vi "Process.vi"(8 "error in":errorcluster, 11 "Generator":refnum<class "Generator.lvclass">) -> (0 "error out":errorcluster, 3 "Generator out":refnum<class "Generator.lvclass">)   [LabVIEW 2019, in "Generator.lvclass"]
uses:
  Generator.lvclass
  C:/Program Files/National Instruments/LabVIEW 2019/vi.lib/JKI/JKI SMO/SMO/SMO.lvclass
  Generator.lvclass/Generator.ctl
  typedefs/Generator.State--enum.ctl
  <vilib>/JKI/JKI SMO/SMO/SMO.lvclass/SMO.ctl
  929f499e-e52d-49ce-8fd4-6eb7de19c2ac.vi
  9c9ff3dc-a17c-4e79-91bb-522cf085dd97.vi
  7f9fb2fb-b452-4165-b08b-fdce49342378.vi
  <vilib>/JKI/JKI SMO/SMO/Private/ReftoDVR--SMO.vi
  <vilib>/dlg_ctls.llb/Space Constant.vi
  <vilib>/AdvancedString/1D String Array to Delimited String.vi
  <vilib>/JDP Science/JSONtext/Variant to JSON Text.vi
  <vilib>/JDP Science/JSONtext/LVClass Serializer/JSONtext LVClass Serializer.lvclass
  <vilib>/JKI/JKI SMO/SMO/SMO.lvclass
  <userlib>/LevyLab/Debug/Debug.lvlib
panel:
  out "time (ms)":dbl=1.0 min=1.0 format="%#_6p"
  out "String 3":string
  in  "timeout (ms)":i32=10 min=1
  out "String 2":string
  out "String":string
  # "Generator"
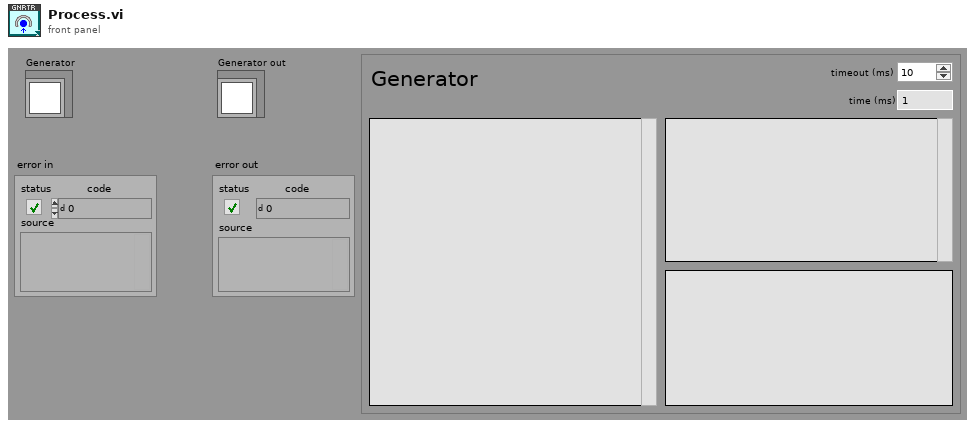
[diagram p1: front panel]
types:
  T1 = typedef "Generator.lvclass/Generator.State--enum.ctl" = enum16{"idle", "started"}
  T2 = enum32{"invalid app kind", "Development System", "Run Time System", "Student Edition", "Embedded LabVIEW", "Evaluation", "Custom"}
  T3 = enum32{"Invalid", "Standard", "Closed", "Hidden", "Minimized", "Maximized"}
  T4 = cluster{"Core":cluster{"Current VI Reference":refnum<vi>, "Close Panel on Exit?":bool, "Last Error":cluster{"error":errorcluster, "previous state":string, "remaining states":string}, "Shutdown?":bool}, "SMO":refnum<class "Generator.lvclass">, "state":T1}
  T5 = typedef "Generator.lvclass/AO.Channel--Cluster--Array.ctl" = T6[]
  T6 = typedef "Generator.lvclass/AO.Channel--Cluster.ctl" = cluster{"Enable?":bool, "Channel":i32, "Amplitude":dbl, "Offset":dbl, "Frequency":dbl, "Phase":dbl, "Function":T7, "Sweeping?":bool, "Limit AC?":bool, "Limit DC?":bool, "Duty Cycle?":bool, "Duty Cycle":dbl}
  T7 = typedef "Generator.lvclass/AO.Channel.Function--Enum.ctl" = enum16{"sine", "square", "triangle", "saw"}
  T8 = typedef "Generator.lvclass/REF.Channel--Cluster--Array.ctl" = T9[]
  T9 = typedef "Generator.lvclass/REF.Channel--Cluster.ctl" = cluster{"Enable?":bool, "Channel":i32, "Frequency":dbl, "Phase":dbl, "TC":dbl, "Roll-Off":i32}
  T10 = typedef "Generator.lvclass/Sweep.Channel--Cluster--Array.ctl" = T11[]
  T11 = typedef "Generator.lvclass/Sweep.Channel--Cluster.ctl" = cluster{"Enable?":bool, "Channel":u16, "Start":dbl, "End":dbl, "Pattern":T12, "Table":dbl[]}
  T12 = typedef "Generator.lvclass/Sweep.Pattern--Enum.ctl" = enum16{"Ramp /", "Ramp /\\", "Smooth Ramp _/", "Smooth Ramp _/\\_", "Table"}
  T13 = typedef "Generator.lvclass/Generator.Command--enum.ctl" = enum16{"start", "stop", "start sweep", "stop sweep"}
  T14 = cluster{"Current VI Reference":refnum<vi>, "Close Panel on Exit?":bool, "Last Error":cluster{"error":errorcluster, "previous state":string, "remaining states":string}, "Shutdown?":bool}
  T15 = typedef "Debug.lvlib/Attribute.Debug.lvclass/DebugBehavior.ctl" = enum16{"Normal", "Debug"}
  T16 = typedef "SMO.lvclass/Protected Events.ctl" = cluster{"StopProcesses":refnum<user-event>, "AbortProcesses":refnum<user-event>, "Config Changed":refnum<user-event>, "Dependency":refnum<user-event>}
  T17 = typedef "Generator.lvclass/PrivateEvents--Cluster.ctl" = cluster{"Message":refnum<user-event>, "Sampling":refnum<user-event>, "AOchannel":refnum<user-event>, "REFchannel":refnum<user-event>, "Sweep":refnum<user-event>, "Command":refnum<user-event>, "WaveformQueues":refnum<user-event>}
  T18 = typedef "Generator.lvclass/Waveforms--Cluster.ctl" = cluster{"AO":waveform(dbl)[], "REF_X":waveform(dbl)[], "REF_Y":waveform(dbl)[]}
  T19 = typedef "Generator.lvclass/Generator.Sweep Status--enum.ctl" = enum16{"idle", "initializing", "waiting", "sweeping", "stopping"}
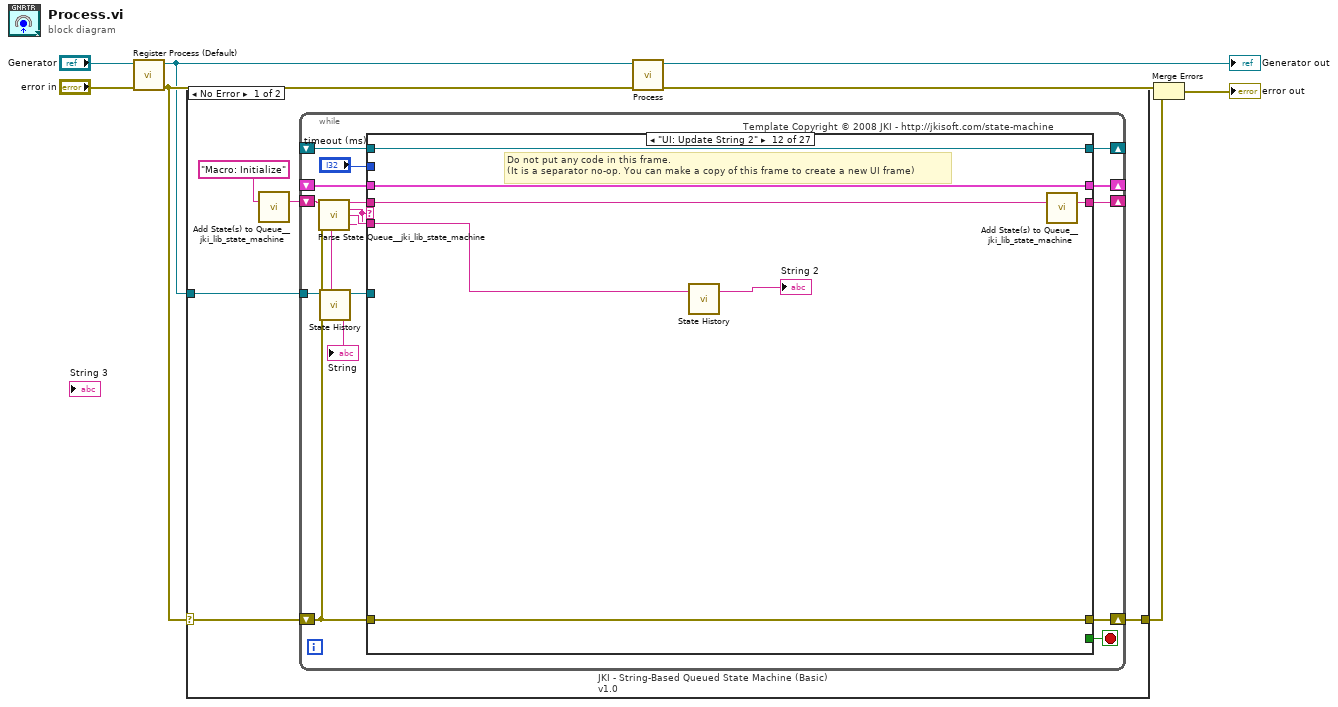
[diagram p0: block diagram]
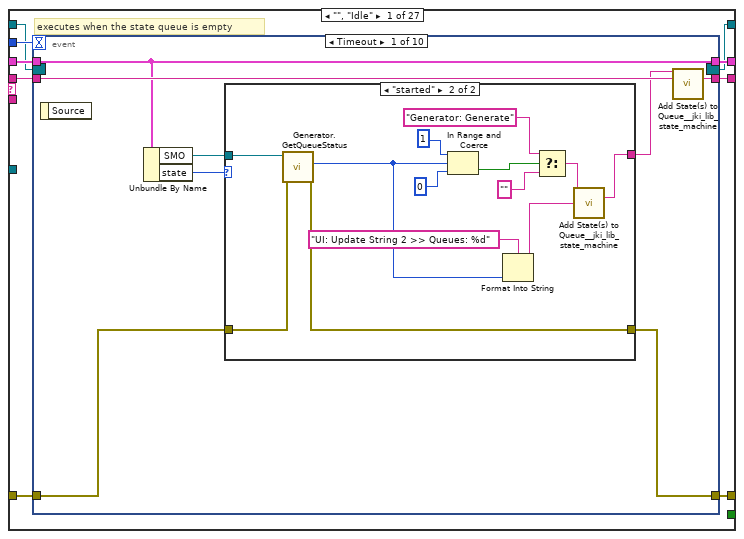
[diagram p2: hidden frame]
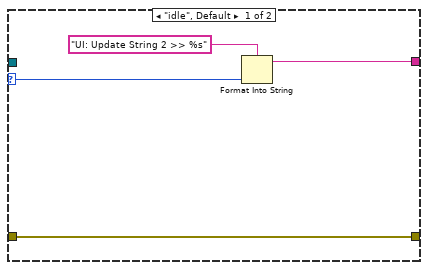
[diagram p3: hidden frame]
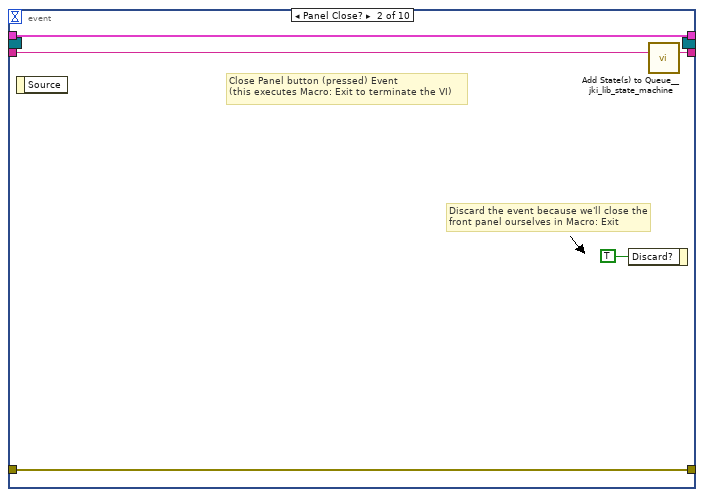
[diagram p4: hidden frame]
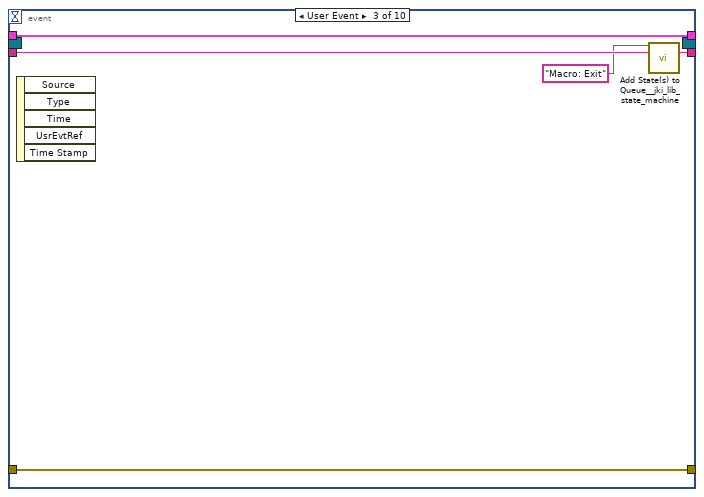
[diagram p5: hidden frame]
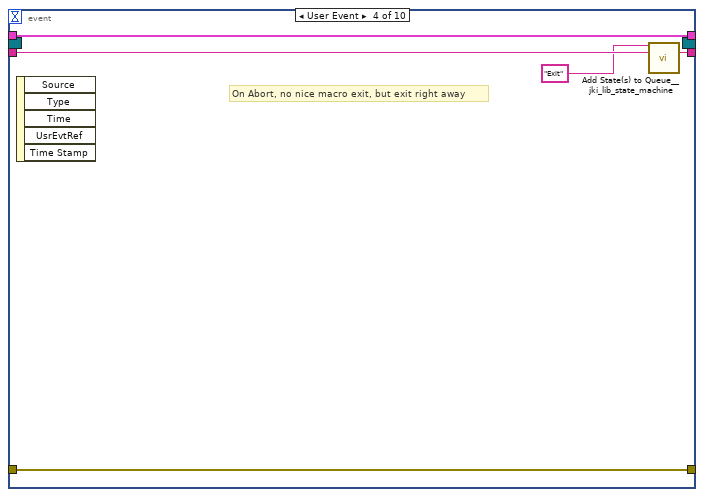
[diagram p6: hidden frame]
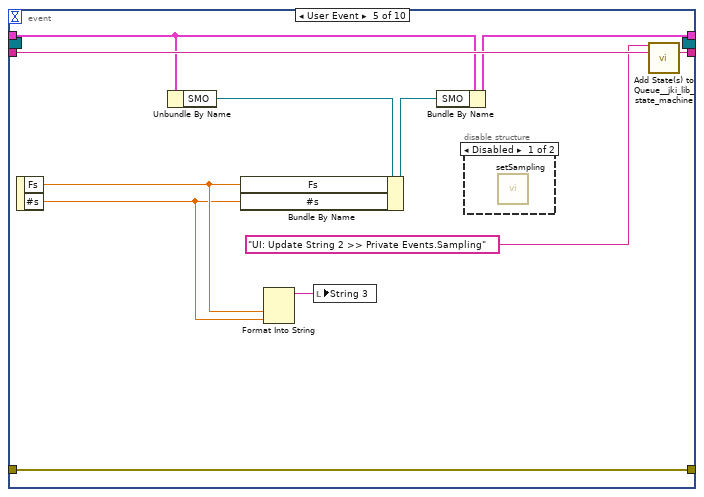
[diagram p7: hidden frame]
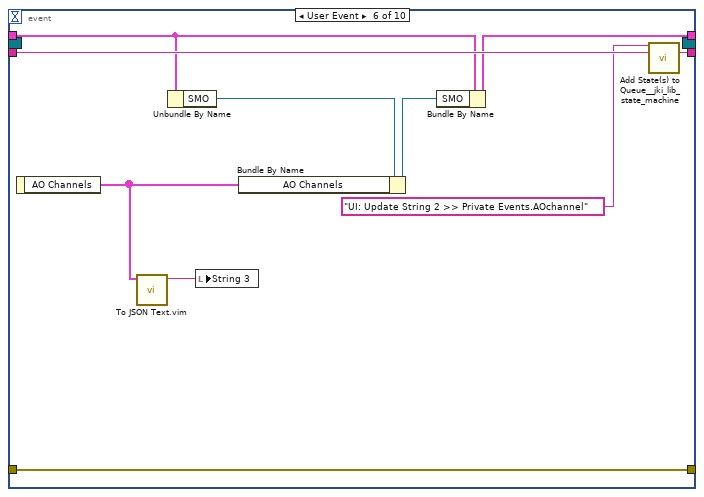
[diagram p9: hidden frame]
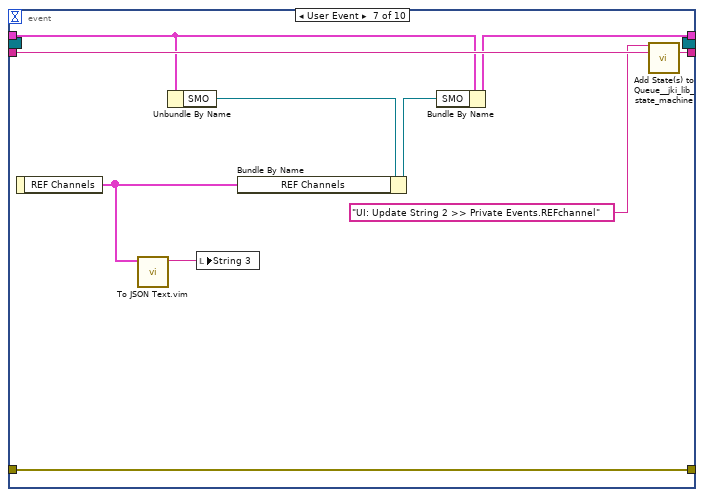
[diagram p10: hidden frame]
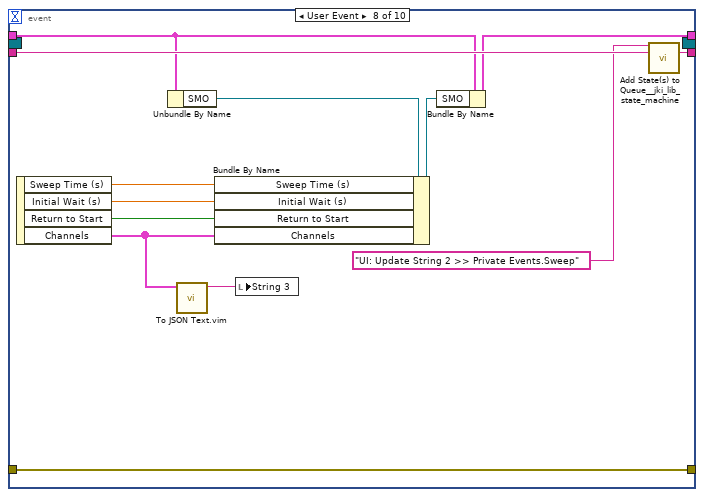
[diagram p11: hidden frame]
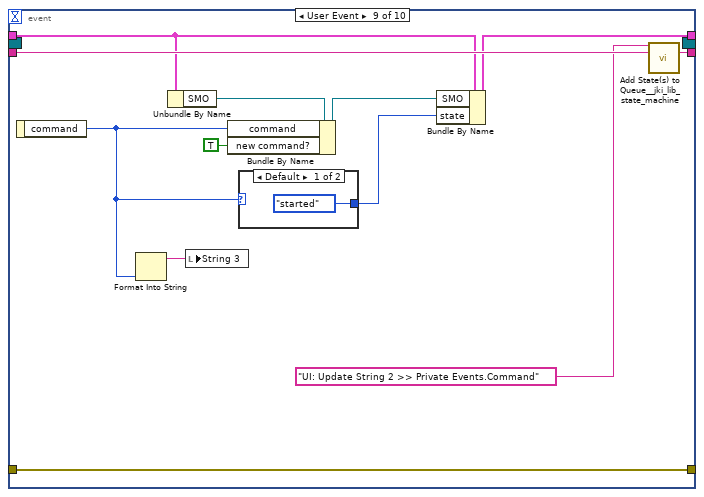
[diagram p12: hidden frame]
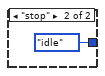
[diagram p13: hidden frame]
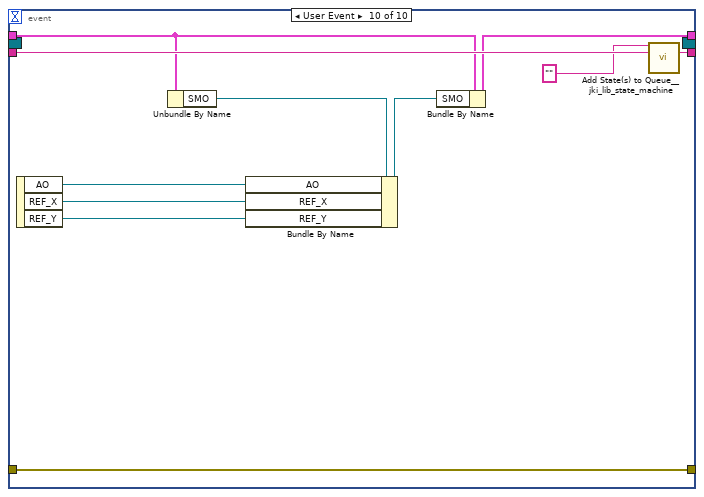
[diagram p14: hidden frame]
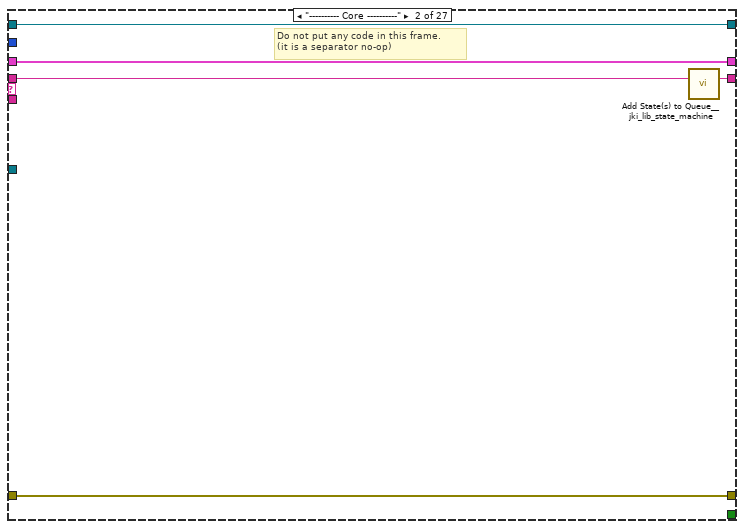
[diagram p15: hidden frame]
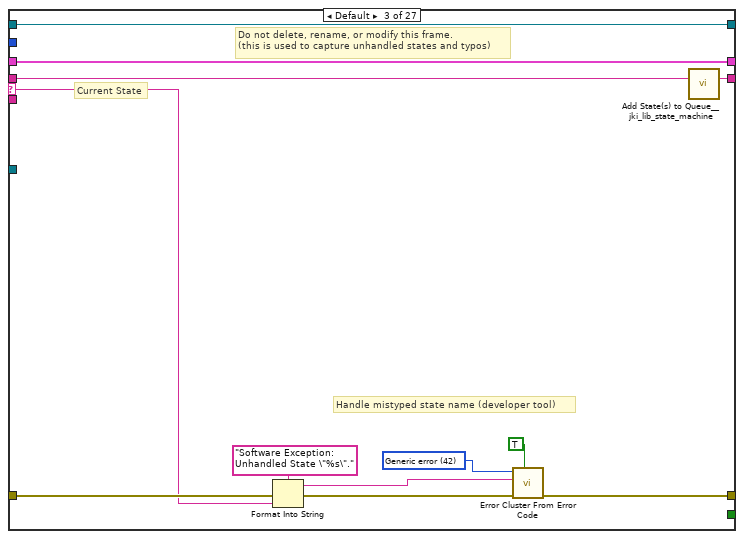
[diagram p16: hidden frame]
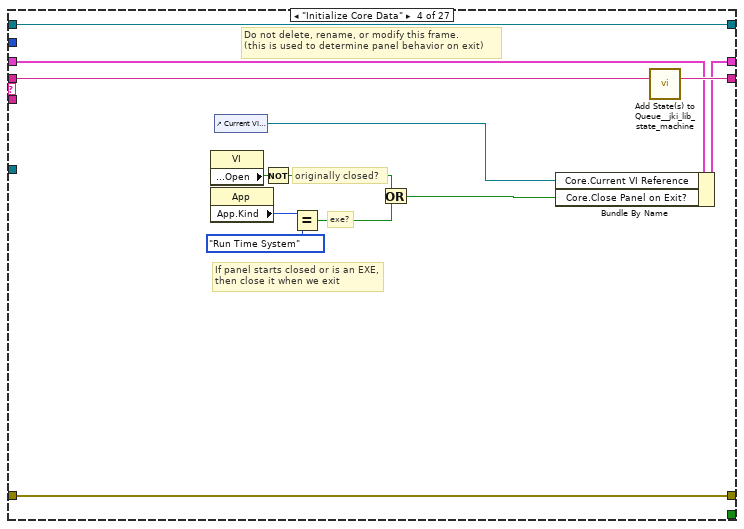
[diagram p17: hidden frame]
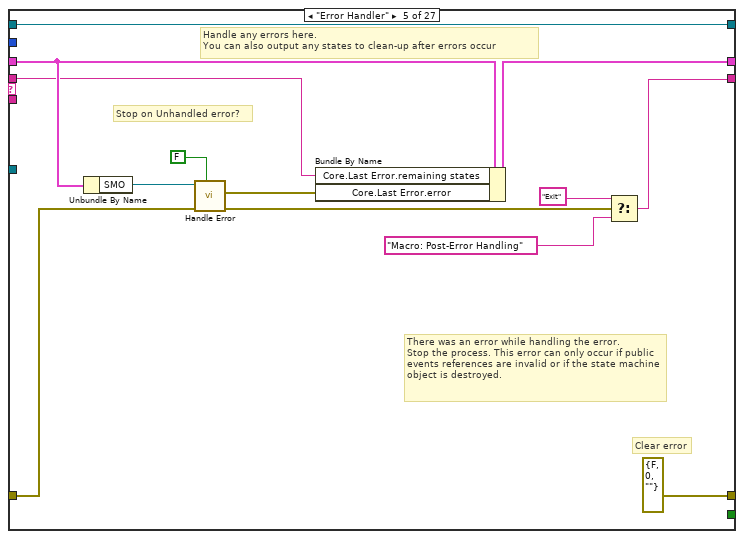
[diagram p18: hidden frame]
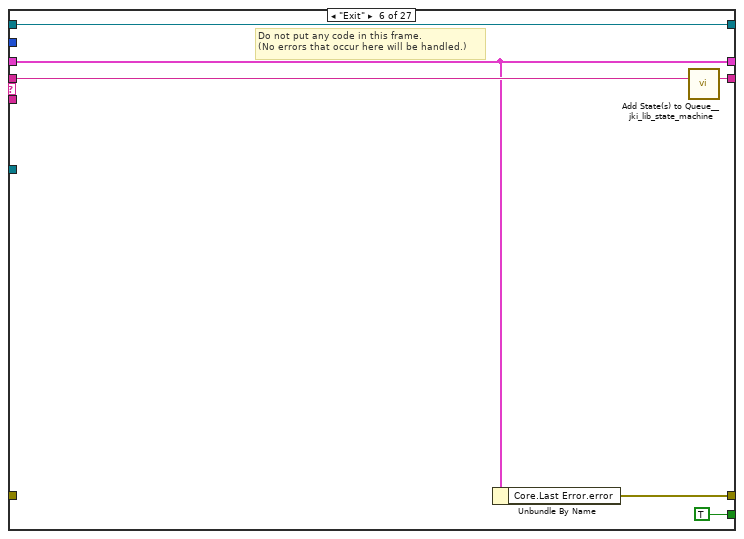
[diagram p19: hidden frame]
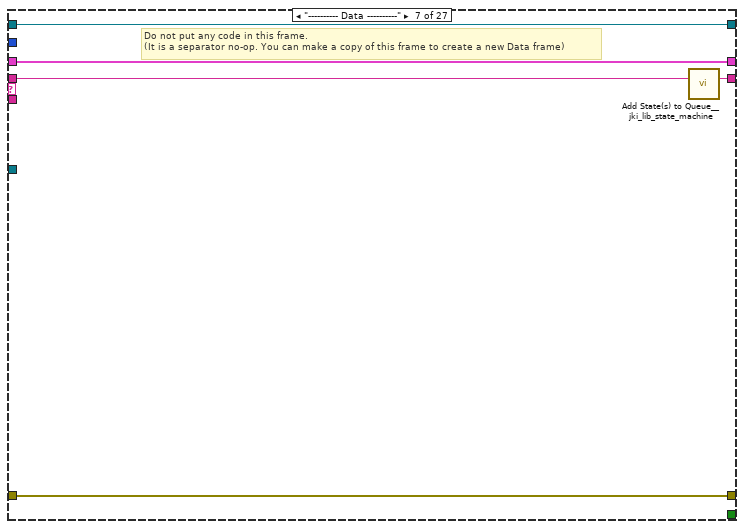
[diagram p20: hidden frame]
diagram:
  n1 = call <vilib>:"Register Process (Default).vi"("error in (no error)"="error in", "SMO"="Generator") -> ("error out"=w4:errorcluster, "SelfRef"=w3:refnum<class "Generator.lvclass">)  [unwired: 8 in]
  n2 = case shown="No Error" w4 {
    selector: w4 -> [w12 w441]
    tunnel: w3 -> [w13 _]
    tunnel: [w11 w441] -> w2
    frame No Error {
      n3 = call <vilib>:"Add State(s) to Queue__jki_lib_state_machine.vi"("State(s) in (\"\")"="Macro: Initialize") -> ("States Out"=w9:string)  [unwired: 14 in]
      n4 = while "JKI - String-Based Queued State Machine (Basic) v1.0" {
        shift-right: [w23] -> _
        shift-left: _ -> [w22]
        shift-right: [w26] -> w11
        shift-left: w12 -> [w21]
        shift-right: [w25] -> _
        shift-left: w9 -> [w27]
        tunnel: w13 -> [w16]
        shift-right: [w20] -> _
        shift-left: _ -> [w19]
        stop <- w24 stop-if-true
        # "Template Copyright © 2008 JKI - http://jkisoft.com/state-machine"
        n5 = call <vilib>:"Parse State Queue__jki_lib_state_machine.vi"("State Queue"=w27, "Error In (no error)"=w21) -> ("Remaining States"=w29:string, "Current State"=w15:string, "Arguments"=w28:string)  [unwired: 11 in]
        n6 = call <userlib>:"State History.vi"("Current State"=w15, "SMO"=w16) -> ("SMO"=w17:refnum<class "Generator.lvclass">, "History"=→"String":string)  [unwired: 8 in]
        n7 = case shown="\"UI: Update String 2\"" w15 {
          selector: w15 -> [_ _ w154 _ _ _ _ _ _ _ _ _ w238 _ _ _ _ _ _ _ _ _ _ _ _ _ _]
          tunnel: w29 -> [w38 w152 w158 w177 w179 w196 w201 w209 w216 w221 w227 w234 w237 w257 w273 w305 w314 w320 w346 w363 w368 w379 w384 w397 w403 w410 w430]
          tunnel: w28 -> [_ _ _ _ _ _ _ _ _ _ _ w228 w235 w251 w269 _ _ _ _ _ _ _ _ _ _ _ _]
          tunnel: w22 -> [w36 w149 w156 w168 w188 w192 w198 _ w211 w218 w225 w231 w248 w255 w271 w302 w310 w317 w338 w353 w365 w376 w381 w395 w401 w406 w423]
          tunnel: [w35 w150 w160 w174 errorcluster {"status"=FALSE, "code"=0, "source"=""} ("error out") w191 w199 w204 w212 w219 w223 w232 w249 w252 w266 w303 w312 w316 w344 w361 w366 w370 w382 w388 w399 w404 w424] -> w26
          tunnel: w21 -> [w34 w150 w159 w174 w185 _ w199 w204 w213 w219 w222 w232 w249 w253 w267 w303 w312 w315 w344 w361 w366 w371 w382 w391 w399 w404 w426]
          tunnel: [w37 w151 w157 w176 w178 w195 w200 w208 w215 w220 w226 w233 w250 w256 w272 w304 w313 w329 w345 w362 w367 w378 w383 w396 w402 w409 w429] -> w25
          tunnel: [_ _ _ _ _ TRUE _ _ _ _ _ _ _ _ _ _ _ _ _ _ _ _ _ _ _ _ _] -> w24
          tunnel: [w33 w149 w156 w175 w187 w192 w198 w207 w211 w218 w225 w231 w248 w255 w271 w302 w310 w318 w342 w352 w365 w376 w381 w395 w401 w407 w427] -> w23
          tunnel: "timeout (ms)" -> [w32 _ _ _ _ _ _ _ _ _ _ _ _ _ _ _ _ _ _ _ _ _ _ _ _ _ _]
          tunnel: w17 -> [_ _ _ _ _ _ _ w203 _ _ _ _ _ _ _ _ _ _ _ _ _ _ _ _ _ _ _]
          tunnel: [w30 w148 w153 w165 w190 w193 w197 w206 w210 w217 w224 w230 w247 w254 w270 w301 w311 w328 w343 w355 w364 w377 w380 w393 w400 w408 w428] -> w20
          tunnel: w19 -> [w31 w148 w153 w165 w190 w193 w197 w206 w210 w217 w224 w230 w247 w254 w270 w301 w311 w328 w343 w355 w364 w377 w380 _ w400 w408 w428]
          frame "", "Idle" {
            # "executes when the state queue is empty"
            n8 = event shown="[0] Timeout" {
              selector: w31 -> [_ _ _ _ _ _ _ _ _ _]
              dyn-events: [_ _ _ _ _ _ _ _ _ _] -> w30
              timeout: w32 -> [_ _ _ _ _ _ _ _ _ _]
              tunnel: w38 -> [w46 w68 w73 w78 w89 w99 w109 w122 w134 w147]
              tunnel: [w45 w67 w72 w77 w88 w98 w108 w121 w133 w146] -> w37
              tunnel: w36 -> [w44 w64 w70 w75 w83 w92 w103 w114 w127 w139]
              tunnel: [w40 w66 w71 w76 w87 w97 w107 w120 w132 w145] -> w35
              tunnel: w34 -> [w41 w66 w71 w76 w87 w97 w107 w120 w132 w145]
              tunnel: [w44 w64 w70 w75 w84 w93 w104 w115 w128 w140] -> w33
              event Timeout {
                n9 = event-data() -> ()  [unwired: 1 in, 1 out]
                n10 = Unbundle By Name(w44) -> ("SMO"=w43:refnum<class "Generator.lvclass">, "state"=w39:T1)
                n11 = case shown="\"started\"" w39 {
                  selector: w39 -> [w49 _]
                  tunnel: w43 -> [_ w63]
                  tunnel: [w47 w52] -> w42
                  tunnel: w41 -> [w50 w56]
                  tunnel: [w50 w55] -> w40
                  frame "idle", Default {
                    n12 = Format Into String(format string="UI: Update String 2 >> %s" ("f"), w49) -> (resulting string=w47:string)  [unwired: 2 in, 1 out]
                  }
                  frame "started" {
                    n13 = call "Generator.GetQueueStatus.vi"("error in (no error)"=w56, "Generator in"=w63) -> ("error out"=w55:errorcluster, "# elements"=w60:i32)  [unwired: 7 in, 1 out]
                    n14 = In Range and Coerce(upper limit=1 ("x"), x=w60, lower limit=0 ("x")) -> (In Range?=w59:bool)  [unwired: 1 out]
                    n15 = Format Into String(format string="UI: Update String 2 >> Queues: %d" ("f"), w60) -> (resulting string=w54:string)  [unwired: 2 in, 1 out]
                    n16 = Select(t="Generator: Generate", s=w59, f="") -> (s? t:f=w53:string)
                    n17 = call <vilib>:"Add State(s) to Queue__jki_lib_state_machine.vi"("State(s) in Front (\"\")"=w53, "State(s) at Back (\"\")"=w54) -> ("States Out"=w52:string)  [unwired: 13 in]
                  }
                }
                n18 = call <vilib>:"Add State(s) to Queue__jki_lib_state_machine.vi"("State(s) in Front (\"\")"=w42, "State(s) in (\"\")"=w46) -> ("States Out"=w45:string)  [unwired: 13 in]
              }
              event Panel Close? {
                # "Discard the event because we'll close the front panel ourselves in Macro: Exit"
                # "Close Panel button (pressed) Event\n(this executes Macro: Exit to terminate the VI)"
                n19 = event-data() -> ()  [unwired: 1 in, 1 out]
                n20 = event-data("Discard?"=TRUE) -> ()  [unwired: 1 in, 1 out]
                n21 = call <vilib>:"Add State(s) to Queue__jki_lib_state_machine.vi"("State(s) in (\"\")"=w68) -> ("States Out"=w67:string)  [unwired: 14 in]
              }
              event User Event {
                n22 = event-data() -> ()  [unwired: 1 in, 5 out]
                n23 = call <vilib>:"Add State(s) to Queue__jki_lib_state_machine.vi"("State(s) in Front (\"\")"="Macro: Exit", "State(s) in (\"\")"=w73) -> ("States Out"=w72:string)  [unwired: 13 in]
              }
              event User Event {
                # "On Abort, no nice macro exit, but exit right away"
                n24 = event-data() -> ()  [unwired: 1 in, 5 out]
                n25 = call <vilib>:"Add State(s) to Queue__jki_lib_state_machine.vi"("State(s) in Front (\"\")"="Exit", "State(s) in (\"\")"=w78) -> ("States Out"=w77:string)  [unwired: 13 in]
              }
              event User Event {
                n26 = event-data() -> ("Fs"=w80:dbl, "#s"=w79:dbl)  [unwired: 1 in]
                n27 = Unbundle By Name(w83) -> ("SMO"=w86:refnum<class "Generator.lvclass">)
                n28 = Bundle By Name(cluster=w86, "Fs"=w80, "#s"=w79) -> (w85:refnum<class "Generator.lvclass">)
                n29 = Format Into String(w80, w79) -> (resulting string=w81:string)  [unwired: 3 in, 1 out]
                n30 = local write "String 3"(w81) -> ()
                n31 = Bundle By Name(cluster=w83, "SMO"=w85) -> (w84:T4)
                n32 = disable-structure shown="Disabled" {
                  frame Disabled {
                    n33 = call "setSampling.vi"() -> ()  [unwired: 10 in, 2 out]
                  }
                  frame Enabled {
                  }
                }
                n34 = call <vilib>:"Add State(s) to Queue__jki_lib_state_machine.vi"("State(s) in Front (\"\")"="UI: Update String 2 >> Private Events.Sampling", "State(s) in (\"\")"=w89) -> ("States Out"=w88:string)  [unwired: 13 in]
              }
              event User Event {
                n35 = event-data() -> ("AO Channels"=w91:T5)  [unwired: 1 in]
                n36 = call "To JSON Text.vim"("Anything"=w91) -> ("<JSON>"=w90:string)  [unwired: 9 in, 1 out]
                n37 = Unbundle By Name(w92) -> ("SMO"=w95:refnum<class "Generator.lvclass">)
                n38 = local write "String 3"(w90) -> ()
                n39 = Bundle By Name(cluster=w95, "AO Channels"=w91) -> (w94:refnum<class "Generator.lvclass">)
                n40 = Bundle By Name(cluster=w92, "SMO"=w94) -> (w93:T4)
                n41 = call <vilib>:"Add State(s) to Queue__jki_lib_state_machine.vi"("State(s) in Front (\"\")"="UI: Update String 2 >> Private Events.AOchannel", "State(s) in (\"\")"=w99) -> ("States Out"=w98:string)  [unwired: 13 in]
              }
              event User Event {
                n42 = event-data() -> ("REF Channels"=w100:T8)  [unwired: 1 in]
                n43 = call "To JSON Text.vim"("Anything"=w100) -> ("<JSON>"=w101:string)  [unwired: 9 in, 1 out]
                n44 = Unbundle By Name(w103) -> ("SMO"=w106:refnum<class "Generator.lvclass">)
                n45 = local write "String 3"(w101) -> ()
                n46 = Bundle By Name(cluster=w106, "REF Channels"=w100) -> (w105:refnum<class "Generator.lvclass">)
                n47 = Bundle By Name(cluster=w103, "SMO"=w105) -> (w104:T4)
                n48 = call <vilib>:"Add State(s) to Queue__jki_lib_state_machine.vi"("State(s) in Front (\"\")"="UI: Update String 2 >> Private Events.REFchannel", "State(s) in (\"\")"=w109) -> ("States Out"=w108:string)  [unwired: 13 in]
              }
              event User Event {
                n49 = event-data() -> ("Sweep Time (s)"=w118:dbl, "Initial Wait (s)"=w112:dbl, "Return to Start"=w113:bool, "Channels"=w110:T10)  [unwired: 1 in]
                n50 = Unbundle By Name(w114) -> ("SMO"=w117:refnum<class "Generator.lvclass">)
                n51 = call "To JSON Text.vim"("Anything"=w110) -> ("<JSON>"=w111:string)  [unwired: 9 in, 1 out]
                n52 = Bundle By Name(cluster=w117, "Sweep Time (s)"=w118, "Initial Wait (s)"=w112, "Return to Start"=w113, "Channels"=w110) -> (w116:refnum<class "Generator.lvclass">)
                n53 = local write "String 3"(w111) -> ()
                n54 = Bundle By Name(cluster=w114, "SMO"=w116) -> (w115:T4)
                n55 = call <vilib>:"Add State(s) to Queue__jki_lib_state_machine.vi"("State(s) in Front (\"\")"="UI: Update String 2 >> Private Events.Sweep", "State(s) in (\"\")"=w122) -> ("States Out"=w121:string)  [unwired: 13 in]
              }
              event User Event {
                n56 = event-data() -> ("command"=w124:T13)  [unwired: 1 in]
                n57 = Format Into String(w124) -> (resulting string=w125:string)  [unwired: 3 in, 1 out]
                n58 = Unbundle By Name(w127) -> ("SMO"=w130:refnum<class "Generator.lvclass">)
                n59 = local write "String 3"(w125) -> ()
                n60 = Bundle By Name(cluster=w130, "command"=w124, "new command?"=TRUE) -> (w129:refnum<class "Generator.lvclass">)
                n61 = case shown="Default" w124 {
                  tunnel: [Generator.State--enum."started" ("state") Generator.State--enum."idle" ("state")] -> w126
                  frame Default {
                  }
                  frame "stop" {
                  }
                }
                n62 = Bundle By Name(cluster=w127, "SMO"=w129, "state"=w126) -> (w128:T4)
                n63 = call <vilib>:"Add State(s) to Queue__jki_lib_state_machine.vi"("State(s) in Front (\"\")"="UI: Update String 2 >> Private Events.Command", "State(s) in (\"\")"=w134) -> ("States Out"=w133:string)  [unwired: 13 in]
              }
              event User Event {
                n64 = event-data() -> ("AO"=w143:refnum<queue>, "REF_X"=w138:refnum<queue>, "REF_Y"=w137:refnum<queue>)  [unwired: 1 in]
                n65 = Unbundle By Name(w139) -> ("SMO"=w142:refnum<class "Generator.lvclass">)
                n66 = Bundle By Name(cluster=w142, "AO"=w143, "REF_X"=w138, "REF_Y"=w137) -> (w141:refnum<class "Generator.lvclass">)
                n67 = Bundle By Name(cluster=w139, "SMO"=w141) -> (w140:T4)
                n68 = call <vilib>:"Add State(s) to Queue__jki_lib_state_machine.vi"("State(s) in Front (\"\")"="", "State(s) in (\"\")"=w147) -> ("States Out"=w146:string)  [unwired: 13 in]
              }
            }
          }
          frame "---------- Core ----------" {
            # "Do not put any code in this frame.\n(it is a separator no-op)"
            n69 = call <vilib>:"Add State(s) to Queue__jki_lib_state_machine.vi"("State(s) in (\"\")"=w152) -> ("States Out"=w151:string)  [unwired: 14 in]
          }
          frame Default {
            w163 = 42 items=["No error", "Argument error", "Memory is full", "Out of zone", "End of file", "File already open", "Generic file I/O error", "File not found", "File permission error", "Disk is full", "Duplicate path", "Too many files open", "System feature not enabled", "Resource file not found", "Cannot add resource", "Resource not found", "Image not found", "Image memory error", "Pen does not exist", "Config type invalid", "Config token not found", "Config parse error", "Config memory error", "Bad external code format", "Bad external code offset", "External code not present", "Null window", "Destroy window error", "Null menu", "Print aborted", "Bad print record", "Print driver error", "Windows error during printing", "Memory error during printing", "Print dialog error", "Generic print error", "Invalid device refnum", "Device not found", "Device parameter error", "Device unit error", "Cannot open device", "Device call aborted", "Generic error", "Cancelled by user", "Object ID too low", "Object ID too high", "Object not in heap", "Unknown heap", "Unknown object (invalid DefProc)", "Unknown object (DefProc not in table)", "Message out of range", "Invalid (null) method", "Unknown message", "Manager call not supported", "Bad address", "Network operation in progress", "Network operation timed out", "Connection is busy", "Network attribute not supported", "Network error", "Address in use", "System out of memory", "Connection aborted", "Connection refused", "Not connected", "Already connected", "Connection closed", "Initialization error (interapplication manager)", "Bad occurrence", "Wait on unbound occurrence handler", "Occurrence queue overflow", "Datalog type conflict", "Unused", "Unrecognized type (interapplication manager)", "Memory corrupt", "Failed to make temporary DLL", "Old CIN version", "Drag socket not found", "Failed to load drop-object", "Failed to register OLE object", "Failed to release OLE object", "Format specifier type mismatch", "Unknown format specifier", "Too few format specifiers", "Too many format specifiers", "Scan failed", "Newer CIN version", "Error converting to variant", "Runtime menu error", "Password tampered", "Variant attribute not found", "Incompatible variant data type", "Event data is not available", "Event Store is not present", "Occurrence is not found", "Event Queue is not created", "Event info is not available", "Refnum passed is NULL", "Error retrieving Class GUID", "Error retrieving CoClass GUID", "Error retrieving TypeLib GUID.", "Bad built application magic bytes.", "Specific driver is different from the specific driver associated with the Logical Name.", "There is no session opened to the class driver.", "Max Error", "MAX - Error with config objects", "MAX - Error loading configuration", "MAX - Group not supported"]
            # "Current State"
            # "Do not delete, rename, or modify this frame.\n(this is used to capture unhandled states and typos)"
            # "Handle mistyped state name (developer tool)"
            n70 = Format Into String(format string="Software Exception: Unhandled State \"%s\"." ("message"), error in=w159, w154) -> (resulting string=w162:string, error out=w161:errorcluster)  [unwired: 1 in]
            n71 = call <vilib>:"Error Cluster From Error Code.vi"("show call chain? (False)"=TRUE, "error in (no error)"=w161, "error message (\"\")"=w162, "error code (0)"=w163) -> ("error out"=w160:errorcluster)  [unwired: 5 in]
            n72 = call <vilib>:"Add State(s) to Queue__jki_lib_state_machine.vi"("State(s) in (\"\")"=w158) -> ("States Out"=w157:string)  [unwired: 14 in]
          }
          frame "Initialize Core Data" {
            # "Do not delete, rename, or modify this frame.\n(this is used to determine panel behavior on exit)"
            # "originally closed?"
            # "exe?"
            # "If panel starts closed or is an EXE, then close it when we exit"
            n73 = property class="VI"() -> ("Front Panel.Open"=w173:bool)  [unwired: 2 in, 2 out]
            n74 = property class="App"() -> ("App.Kind"=w172:T2)  [unwired: 2 in, 2 out]
            n75 = control-ref of="Current VI Reference"() -> (w166:refnum<vi>)
            n76 = Not(x=w173) -> (.not. x?=w170:bool)
            n77 = Equal?(x=w172, y=T2."Run Time System" ("Application:Kind")) -> (x = y?=w169:bool)
            n78 = Or(x=w170, y=w169) -> (x .or. y?=w167:bool)
            n79 = Bundle By Name(cluster=w168, "Core.Current VI Reference"=w166, "Core.Close Panel on Exit?"=w167) -> (w175:T4)
            n80 = call <vilib>:"Add State(s) to Queue__jki_lib_state_machine.vi"("State(s) in (\"\")"=w177) -> ("States Out"=w176:string)  [unwired: 14 in]
          }
          frame "Error Handler" {
            # "Stop on Unhandled error?"
            # "There was an error while handling the error.\nStop the process. This error can only occur if public events references are invalid or if the state machine object is destroyed."
            # "Handle any errors here.\nYou can also output any states to clean-up after errors occur"
            # "Clear error"
            n81 = Unbundle By Name(w188) -> ("SMO"=w189:refnum<class "Generator.lvclass">)
            n82 = call-dynamic "Handle Error.vi"("Stop on Unhandled Error (T)"=FALSE, "error in"=w185, "SMO"=w189) -> ("handling error"=w183:errorcluster, "Unhandled error"=w186:errorcluster)  [unwired: 6 in, 1 out]
            n83 = Bundle By Name(cluster=w188, "Core.Last Error.remaining states"=w179, "Core.Last Error.error"=w186) -> (w187:T4)
            n84 = Select(t="Exit", s=w183, f="Macro: Post-Error Handling") -> (s? t:f=w178:string)
          }
          frame "Exit" {
            # "Do not put any code in this frame.\n(No errors that occur here will be handled.)"
            n85 = Unbundle By Name(w192) -> ("Core.Last Error.error"=w191:errorcluster)
            n86 = call <vilib>:"Add State(s) to Queue__jki_lib_state_machine.vi"("State(s) in (\"\")"=w196) -> ("States Out"=w195:string)  [unwired: 14 in]
          }
          frame "---------- Data ----------" {
            # "Do not put any code in this frame.\n(It is a separator no-op. You can make a copy of this frame to create a new Data frame)"
            n87 = call <vilib>:"Add State(s) to Queue__jki_lib_state_machine.vi"("State(s) in (\"\")"=w201) -> ("States Out"=w200:string)  [unwired: 14 in]
          }
          frame "Data: Initialize" {
            w205 = T14 {"Current VI Reference"=refnum, "Close Panel on Exit?"=FALSE, "Last Error"={"error"={"status"=FALSE, "code"=0, "source"=""}, "previous state"="", "remaining states"=""}, "Shutdown?"=FALSE}  # Core
            # "do not delete - used by framework"
            # "Initialize the shift-register data, here.\n(data names are defined by what you wire into the bundle function)"
            n88 = Bundle("Core"=w205, "SMO"=w203, "state"=Generator.State--enum."idle") -> (w207:T4)  [unwired: 1 in]
            n89 = call <vilib>:"Add State(s) to Queue__jki_lib_state_machine.vi"("State(s) in (\"\")"=w209) -> ("States Out"=w208:string)  [unwired: 14 in]
          }
          frame "Data: Cleanup" {
            # "Cleanup any data and references, here.\n(this is called automatically, by the Macro: Exit)"
            n90 = Unbundle By Name(w211) -> ("Core.Current VI Reference"=w214:refnum<vi>)
            n91 = Close Reference(reference=w214, error in (no error)=w213) -> (error out=w212:errorcluster)
            n92 = call <vilib>:"Add State(s) to Queue__jki_lib_state_machine.vi"("State(s) in (\"\")"=w216) -> ("States Out"=w215:string)  [unwired: 14 in]
          }
          frame "---------- UI ----------" {
            # "Do not put any code in this frame.\n(It is a separator no-op. You can make a copy of this frame to create a new UI frame)"
            n93 = call <vilib>:"Add State(s) to Queue__jki_lib_state_machine.vi"("State(s) in (\"\")"=w221) -> ("States Out"=w220:string)  [unwired: 14 in]
          }
          frame "UI: Initialize" {
            # "Initialize the User Interface, here.\n(this is called automatically, by the Macro: Init)"
            n94 = flat-sequence {
              frame #0 {
                # "This is to keep in memory\nfor EXE build"
              }
            }
            n95 = call <userlib>:"Fit VI window to Largest Dec__ogtk.vi"("error in (no error)"=w222) -> ("error out"=w223:errorcluster)  [unwired: 5 in, 1 out]
            n96 = call <vilib>:"Add State(s) to Queue__jki_lib_state_machine.vi"("State(s) in (\"\")"=w227) -> ("States Out"=w226:string)  [unwired: 14 in]
          }
          frame "UI: Update String 2" {
            # "Do not put any code in this frame.\n(It is a separator no-op. You can make a copy of this frame to create a new UI frame)"
            n97 = call <userlib>:"State History.vi"("Current State"=w228) -> ("History"=→"String 2":string)  [unwired: 9 in, 1 out]
            n98 = call <vilib>:"Add State(s) to Queue__jki_lib_state_machine.vi"("State(s) in (\"\")"=w234) -> ("States Out"=w233:string)  [unwired: 14 in]
          }
          frame "UI: Wait" {
            # "UI: Wait.\n(use: \"UI: Wait >> time\" (in ms))"
            n99 = Scan From String(format string="%d", input string=w235, default 1=u32 0 ("default value 1")) -> (output 1=w244:u32)  [unwired: 2 in, 3 out]
            n100 = feedback #1(TRUE ("Triggered")) -> (w241:bool)
            n101 = call <userlib>:"Periodic Trigger__ogtk.vi"("time (ms)"=w244, "reset"=w241) -> ("Triggered"=w242:bool)  [unwired: 11 in, 2 out]
            n102 = feedback-in #1(w242) -> ()
            n103 = call <vilib>:"Build State String with Arguments__JKI_lib_State_Machine.vi"("Arguments (\"\")"=w235, "State"=w238) -> ("State with Arguments"=w240:string)  [unwired: 4 in]
            n104 = Select(t="", s=w242, f=w240) -> (s? t:f=w236:string)
            n105 = call <vilib>:"Add State(s) to Queue__jki_lib_state_machine.vi"("State(s) in Front (\"\")"=w236, "State(s) in (\"\")"=w237) -> ("States Out"=w250:string)  [unwired: 13 in]
          }
          frame "UI: Cursor Set" {
            # "Argument"
            # "Initialize the User Interface, here.\n(this is called automatically, by the Macro: Init)"
            n106 = disable-structure shown="Default" {
              disable-tunnel: w253 -> [w258 w261]
              disable-tunnel: [w258 w260] -> w252
              disable-tunnel: w251 -> [_ w259]
              frame condition #0 {
              }
              frame condition #1 (active) {
                n107 = case shown="\"Idle\", Default" w259 {
                  tunnel: w261 -> [w263 w265]
                  tunnel: [w262 w264] -> w260
                  frame "Idle", Default {
                    n108 = call <vilib>:"Unset Busy.vi"("error in (no error)"=w263) -> ("error out"=w262:errorcluster)  [unwired: 10 in]
                  }
                  frame "Busy" {
                    n109 = call <vilib>:"Set Busy.vi"("error in (no error)"=w265) -> ("error out"=w264:errorcluster)  [unwired: 9 in, 1 out]
                  }
                }
              }
            }
            n110 = call <vilib>:"Add State(s) to Queue__jki_lib_state_machine.vi"("State(s) in (\"\")"=w257) -> ("States Out"=w256:string)  [unwired: 14 in]
          }
          frame "UI: Front Panel State" {
            # "Argument"
            # "Set Front Panel Open or Closed\n(Usage: \"UI: Front Panel State >> Open|Close\")"
            n111 = Unbundle By Name(w271) -> ("Core.Current VI Reference"=w268:refnum<vi>)
            n112 = disable-structure shown="Default" {
              disable-tunnel: w267 -> [w277 w300]
              disable-tunnel: [w276 w300] -> w266
              disable-tunnel: w268 -> [w275 _]
              disable-tunnel: w269 -> [w274 _]
              frame condition #0 (active) {
                n113 = case shown="\"Open\"" w274 {
                  tunnel: w277 -> [w281 w294]
                  tunnel: [w283 w295] -> w276
                  tunnel: w275 -> [w282 w292]
                  frame "Open" {
                    # "Open FP if not open or invalid"
                    n114 = property class="VI"(reference=w282, error in=w281) -> (reference out=w279:refnum<vi>, error out=w280:errorcluster, "FP.State"=w278:T3)
                    n115 = case shown="Default" w278 {
                      tunnel: [w286 w289] -> w283
                      tunnel: w280 -> [w285 w289]
                      tunnel: w279 -> [w284 _]
                      frame Default {
                        n116 = invoke class="VI" method="FP.Open"(reference=w284, error in=w285, "Activate"=TRUE, "State"=T3."Standard") -> (error out=w286:errorcluster)  [unwired: 1 in, 4 out]
                      }
                      frame "Invalid", "Standard" {
                      }
                    }
                  }
                  frame "Close", Default {
                    # "Close FP is not Closed or Invalid"
                    n117 = property class="VI"(reference=w292, error in=w294) -> (reference out=w291:refnum<vi>, error out=w293:errorcluster, "FP.State"=w290:T3)
                    n118 = case shown="Default" w290 {
                      tunnel: [w296 w299] -> w295
                      tunnel: w293 -> [w296 w298]
                      tunnel: w291 -> [_ w297]
                      frame "Invalid", "Closed" {
                      }
                      frame Default {
                        n119 = invoke class="VI" method="FP.Close"(reference=w297, error in=w298) -> (error out=w299:errorcluster)  [unwired: 1 in, 2 out]
                      }
                    }
                  }
                }
              }
              frame condition #1 {
              }
            }
            n120 = call <vilib>:"Add State(s) to Queue__jki_lib_state_machine.vi"("State(s) in (\"\")"=w273) -> ("States Out"=w272:string)  [unwired: 14 in]
          }
          frame "---------- Macro ----------" {
            # "Do not put any code in this frame.\n(It is a separator no-op. You can make a copy of this frame to create a new Macro frame)"
            n121 = call <vilib>:"Add State(s) to Queue__jki_lib_state_machine.vi"("State(s) in (\"\")"=w305) -> ("States Out"=w304:string)  [unwired: 14 in]
          }
          frame "Macro: Initialize" {
            w308 = "UI: Initialize\nUI: Front Panel State >> Close\nMacro: Debug"  # UI: Initialize UI: Front Panel State >> Close Macro: Debug
            # "Initialization Macro\n(This is called once, when the VI starts)"
            n122 = call <vilib>:"Add State(s) to Queue__jki_lib_state_machine.vi"("State(s) in Front (\"\")"="Data: Initialize\nInitialize Core Data\nEvents: Register", "State(s) in (\"\")"="Process: Sync", "State(s) at Back (\"\")"=w308) -> ("States Out"=w307:string)  [unwired: 12 in]
            n123 = call <vilib>:"Add State(s) to Queue__jki_lib_state_machine.vi"("State(s) in Front (\"\")"=w307, "State(s) in (\"\")"=w314) -> ("States Out"=w313:string)  [unwired: 13 in]
          }
          frame "Macro: Debug" {
            # "exe?"
            # "If pane is an EXE, then close it when we exit"
            # "Macro: Debug\n(get debug behavior, determine UI and determine shutdown behavior)"
            n124 = Unbundle By Name(w317) -> ("Core.Close Panel on Exit?"=w322:bool, "SMO"=w327:refnum<class "Generator.lvclass">)
            n125 = property class="App"() -> ("App.Kind"=w325:T2)  [unwired: 2 in, 2 out]
            n126 = Equal?(x=w325, y=T2."Run Time System" ("Application:Kind")) -> (x = y?=w321:bool)
            n127 = call <userlib>:"Get Debug Mode.vi"("error in (no error)"=w315, "SMO"=w327) -> ("error out"=w316:errorcluster, "Behavior"=w326:T15)  [unwired: 7 in, 1 out]
            n128 = case shown="\"Normal\", Default" w326 {
              tunnel: [w330 w332] -> w323
              tunnel: w322 -> [w330 _]
              tunnel: w321 -> [_ w334]
              tunnel: [_ "UI: Front Panel State >> Open\nUI: Wait >> 1000"] -> w319
              frame "Normal", Default {
                # "respect core.close"
              }
              frame "Debug" {
                # "keep panel open\nunless exe"
                n129 = Or(x=w334, y=FALSE) -> (x .or. y?=w332:bool)
              }
            }
            n130 = Bundle By Name(cluster=w317, "Core.Close Panel on Exit?"=w323) -> (w318:T4)
            n131 = call <vilib>:"Add State(s) to Queue__jki_lib_state_machine.vi"("State(s) in Front (\"\")"=w319, "State(s) in (\"\")"=w320) -> ("States Out"=w329:string)  [unwired: 13 in]
          }
          frame "Macro: Post-Error Handling" {
            # "Clear Last Error?"
            n132 = Unbundle By Name(w338) -> ("Core.Last Error.remaining states"=w336:string, "Core.Shutdown?"=w337:bool)
            n133 = Unbundle By Name(w338) -> ("Core.Last Error.error"=w341:errorcluster)
            n134 = case shown="False" FALSE {
              tunnel: w341 -> [w350 _]
              tunnel: [w350 _] -> w340
              frame False {
              }
              frame True {
              }
            }
            n135 = case shown="True" w337 {
              tunnel: w336 -> [w347 w349]
              tunnel: [w347 w348] -> w335
              frame False {
                # "These are the remaining states (at the moment the error occured). States can be altered according to business logic."
                # "NOT SHUTTING DOWN"
              }
              frame True {
                # "Developer can decide to alter the states but should be aware that during the shutdown process, there are certain states that must be run for the SMO to properly shut itself (and this process) down. As such, one can add states to perform additional clean-ups, but should append the remaining state to be executed."
                # "SHUTTING DOWN"
                n136 = call <vilib>:"Add State(s) to Queue__jki_lib_state_machine.vi"("State(s) in (\"\")"=w349) -> ("States Out"=w348:string)  [unwired: 14 in]
              }
            }
            n137 = Bundle By Name(cluster=w338, "Core.Last Error.error"=w340) -> (w342:T4)
            n138 = call <vilib>:"Add State(s) to Queue__jki_lib_state_machine.vi"("State(s) in Front (\"\")"=w335, "State(s) in (\"\")"=w346) -> ("States Out"=w345:string)  [unwired: 13 in]
          }
          frame "Macro: Exit" {
            # "Exit Macro\n(This is called once, when the VI exits)"
            n139 = Unbundle By Name(w353) -> ("Core.Close Panel on Exit?"=w360:bool)
            n140 = Bundle By Name(cluster=w353, "Core.Shutdown?"=TRUE) -> (w352:T4)
            n141 = Select(t="UI: Front Panel State >> Close", s=w360, f="") -> (s? t:f=w357:string)
            n142 = call <vilib>:"Add State(s) to Queue__jki_lib_state_machine.vi"("State(s) in (\"\")"=w357, "State(s) at Back (\"\")"="Data: Cleanup\nEvents: Unregister\nProcess: Sync\nExit") -> ("States Out"=w356:string)  [unwired: 13 in]
            n143 = call <vilib>:"Add State(s) to Queue__jki_lib_state_machine.vi"("State(s) in Front (\"\")"=w356, "State(s) in (\"\")"=w363) -> ("States Out"=w362:string)  [unwired: 13 in]
          }
          frame "---------- Process ----------" {
            # "Template Separator\n(You can make a copy of, or modify, this frame)"
            n144 = call <vilib>:"Add State(s) to Queue__jki_lib_state_machine.vi"("State(s) in (\"\")"=w368) -> ("States Out"=w367:string)  [unwired: 14 in]
          }
          frame "Process: Sync" {
            n145 = Unbundle By Name(w376) -> ("SMO"=w372:refnum<class "Generator.lvclass">)
            n146 = call <vilib>:"WaitOnProcessSync.vi"("error in (no error)"=w371, "SMO"=w372) -> ("error out"=w370:errorcluster, "Don't run?"=w375:bool)  [unwired: 7 in, 1 out]
            n147 = Select(t="Data: Cleanup\nEvents: Unregister\nExit", s=w375, f="") -> (s? t:f=w369:string)
            n148 = call <vilib>:"Add State(s) to Queue__jki_lib_state_machine.vi"("State(s) in Front (\"\")"=w369, "State(s) in (\"\")"=w379) -> ("States Out"=w378:string)  [unwired: 13 in]
          }
          frame "---------- Events ----------" {
            # "Template Separator\n(You can make a copy of, or modify, this frame)"
            n149 = call <vilib>:"Add State(s) to Queue__jki_lib_state_machine.vi"("State(s) in (\"\")"=w384) -> ("States Out"=w383:string)  [unwired: 14 in]
          }
          frame "Events: Register" {
            n150 = Unbundle By Name(w395) -> ("SMO"=w392:refnum<class "Generator.lvclass">)
            n151 = call <vilib>:"GetProtectedEvents.vi"("error in (no error)"=w391, "SMO"=w392) -> ("error out"=w390:errorcluster, "SMO Protected Events"=w394:T16, "SMO out"=w387:refnum<class "Generator.lvclass">)  [unwired: 7 in]
            n152 = call "Generator.GetPrivateEvents.vi"("Generator"=w387) -> ("error out"=w385:errorcluster, "Generator Private Events"=w386:T17)  [unwired: 8 in, 1 out]
            n153 = register-events(w394, w386) -> (reference out=w393:refnum<event-registration>, error out=w389:errorcluster)  [unwired: 2 in]
            n154 = call <vilib>:"Add State(s) to Queue__jki_lib_state_machine.vi"("State(s) in (\"\")"=w397) -> ("States Out"=w396:string)  [unwired: 14 in]
            n155 = Merge Errors(w385, w390, w389) -> (w388:errorcluster)
          }
          frame "Events: Unregister" {
            n156 = Unregister For Events(event registration refnum=w400, error in=w399) -> (error out=w398:errorcluster)
            n157 = call <vilib>:"Clear Errors.vi"("error in (no error)"=w398) -> ()  [unwired: 5 in, 2 out]
            n158 = call <vilib>:"Add State(s) to Queue__jki_lib_state_machine.vi"("State(s) in (\"\")"=w403) -> ("States Out"=w402:string)  [unwired: 14 in]
          }
          frame "--------- Generator ---------" {
            # "Section Separator\n(You can make a copy of, or modify, this frame)"
            n159 = Unbundle By Name(w406) -> ("SMO"=w405:refnum<class "Generator.lvclass">)
            n160 = Bundle By Name(cluster=w406, "SMO"=w405) -> (w407:T4)
            n161 = call <vilib>:"Add State(s) to Queue__jki_lib_state_machine.vi"("State(s) in (\"\")"=w410) -> ("States Out"=w409:string)  [unwired: 14 in]
          }
          frame "Generator: Generate" {
            # "T: add wfm to queue\nF: generate user event"
            # "Generator: Generate\n(You can make a copy of, or modify, this frame)"
            n162 = Unbundle By Name(w423) -> ("SMO"=w422:refnum<class "Generator.lvclass">)
            n163 = call "Generate Waveforms.vi"("error in (no error)"=w426, "Generator.lvclass"=w422) -> ("error out"=w419:errorcluster, "Chart"=→"time (ms)":dbl, "Waveforms out"=w421:T18, "Generator.lvclass"=w420:refnum<class "Generator.lvclass">)  [unwired: 5 in, 1 out]
            n164 = case shown="False" TRUE {
              tunnel: w421 -> [w434 w440]
              tunnel: w420 -> [w435 w439]
              tunnel: w419 -> [w432 w438]
              tunnel: [w433 w437] -> w418
              tunnel: [w431 w436] -> w416
              frame False {
                n165 = call "getWaveforms.vi"("error in (no error)"=w432, "Waveforms"=w434, "Generator in"=w435) -> ("error out"=w431:errorcluster, "Generator out"=w433:refnum<class "Generator.lvclass">)  [unwired: 7 in]
              }
              frame True {
                n166 = call "Generator.AddToQueue.vi"("error in (no error)"=w438, "Waveforms"=w440, "Generator in"=w439) -> ("error out"=w436:errorcluster, "Generator out"=w437:refnum<class "Generator.lvclass">)  [unwired: 7 in]
              }
            }
            n167 = Unbundle By Name(w418) -> ("AO Channels"=w417:T5)
            n168 = call "getAOchannels.vi"("error in (no error)"=w416, "AO Channels"=w417, "Generator in"=w418) -> ("error out"=w415:errorcluster, "Generator out"=w414:refnum<class "Generator.lvclass">)  [unwired: 7 in]
            n169 = Unbundle By Name(w414) -> ("sweep status"=w413:T19)
            n170 = call "getSweepStatus.vi"("error in (no error)"=w415, "sweep status"=w413, "Generator in"=w414) -> ("error out"=w424:errorcluster, "Generator out"=w425:refnum<class "Generator.lvclass">)  [unwired: 7 in]
            n171 = Bundle By Name(cluster=w423, "SMO"=w425) -> (w427:T4)
            n172 = call <vilib>:"Add State(s) to Queue__jki_lib_state_machine.vi"("State(s) in (\"\")"=w430) -> ("States Out"=w429:string)  [unwired: 14 in]
          }
        }
      }
    }
    frame Error {
    }
  }
  n173 = call-parent "Process.vi"("error in"=w4, "SMO"=w3) -> ("error out"=w1:errorcluster, "SMO out"=→"Generator out":refnum<class "Generator.lvclass">)  [unwired: 8 in]
  n174 = Merge Errors(w1, w2) -> (→"error out":errorcluster)
